vi "VI Tree - Caraya.vi"   [LabVIEW 2013]
uses:
  classes/Assert/Assert False.vi
  classes/Assert/Assert True.vi
  run-tests/Run Test (Scalar Path).vi
  run-tests/Run Test (VIRefnum Scalar).vi
  run-tests/Run Test (Array Path).vi
  run-tests/Run Test (VIRefnum Array).vi
  run-tests/Run Test (ProjectRefnum).vi
  run-tests/Run Test (Object Array).vi
  run-tests/Run Test (Object).vi
  classes/Assert/Assert.lvclass
  Caraya.lvlib
  classes/Test/Test.lvclass
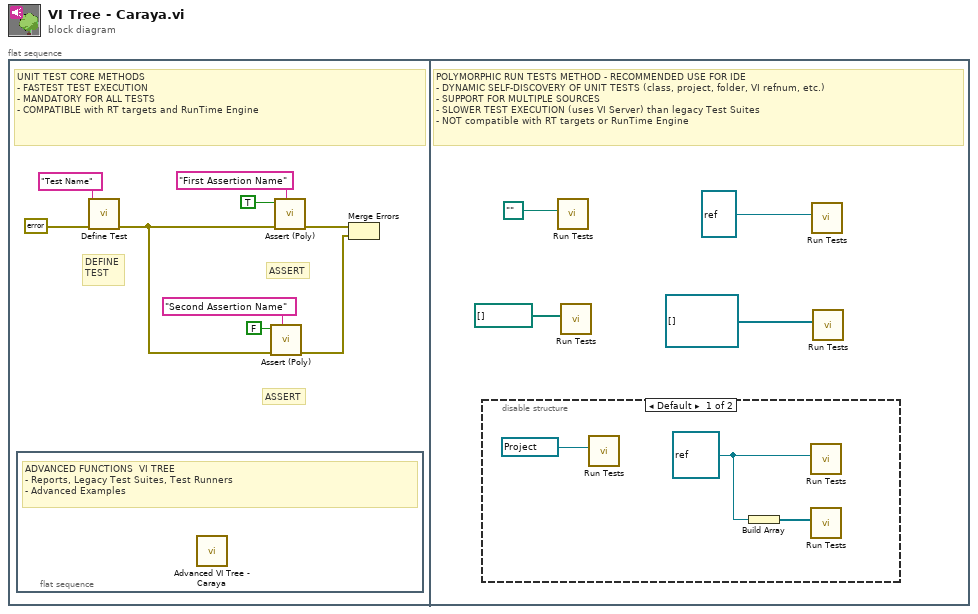
[diagram p0: block diagram]
diagram:
  n1 = flat-sequence {
    frame #0 {
      # "ASSERT"
      # "ASSERT"
      # "DEFINE\nTEST"
      # "UNIT TEST CORE METHODS\n- FASTEST TEST EXECUTION\n- MANDATORY FOR ALL TESTS\n- COMPATIBLE with RT targets and RunTime Engine"
      n2 = flat-sequence {
        frame #0 {
          # "ADVANCED FUNCTIONS  VI TREE\n- Reports, Legacy Test Suites, Test Runners\n- Advanced Examples"
          n3 = call "Advanced VI Tree - Caraya.vi"() -> ()  [unwired: 1 in]
        }
      }
      n4 = call "Define Test.vi"("error in (no error)"=errorcluster {"status"=FALSE, "code"=0, "source"=""}, "Label (VI Title)"="Test Name") -> ("error out"=w5:errorcluster)  [unwired: 9 in]
      n5 = call-poly "Assert (Poly).vi"("Label"="Second Assertion Name" ("Label (VI Title)"), "error in (no error)"=w5, "False?"=FALSE) -> ("error out"=w3:errorcluster)  [unwired: 8 in]
      n6 = call-poly "Assert (Poly).vi"("Label"="First Assertion Name" ("Label (VI Title)"), "error in (no error)"=w5, "True?"=TRUE) -> ("error out"=w4:errorcluster)  [unwired: 8 in]
      n7 = Merge Errors(w4, w3) -> ()  [unwired: 1 out]
    }
    frame #1 {
      # "POLYMORPHIC RUN TESTS METHOD - RECOMMENDED USE FOR IDE\n- DYNAMIC SELF-DISCOVERY OF UNIT TESTS (class, project, folder, VI refnum, etc.)\n- SUPPORT FOR MULTIPLE SOURCES\n- SLOWER TEST EXECUTION (uses VI Server) than legacy Test Suites\n- NOT compatible with RT targets or RunTime Engine"
      n8 = disable-structure shown="Default" {
        frame condition #0 (active) {
          w14 = refnum<class> refnum ("Object")
          n9 = call-poly "Run Tests.vi"("Project Refnum"=refnum<vi> refnum) -> ()  [unwired: 10 in, 1 out]
          n10 = Build Array(w14) -> (w15:refnum<class>[])
          n11 = call-poly "Run Tests.vi"("Object"=w14) -> ()  [unwired: 10 in, 1 out]
          n12 = call-poly "Run Tests.vi"("Objects"=w15) -> ()  [unwired: 10 in, 1 out]
        }
        frame condition #1 {
        }
      }
      n13 = call-poly "Run Tests.vi"("Test Path"=path "") -> ()  [unwired: 10 in, 1 out]
      n14 = call-poly "Run Tests.vi"("Paths"=path[] []) -> ()  [unwired: 10 in, 1 out]
      n15 = call-poly "Run Tests.vi"("VI Refnum"=refnum<vi> refnum) -> ()  [unwired: 10 in, 1 out]
      n16 = call-poly "Run Tests.vi"("VI Refnums"=refnum<vi>[] []) -> ()  [unwired: 10 in, 1 out]
    }
  }
